vi "DistToObstNearwAng.vi"(1 "Boat Point":T1 {"North" format="%#_10f"; "East" format="%#_8f"}, 2 "Segment Point 2":T1 {"North" format="%#_10f"; "East" format="%#_8f"}, 3 "Segment Point 1":T1 {"North" format="%#_10f"; "East" format="%#_8f"}) -> (0 "Distance between boat and segment":dbl)   [LabVIEW 2012]
doc: "Takes in a segment, and a boat point, and returns the distance between the segment and the boat. For obstacle avoidance. To be added: absolute trig angle to segment."
uses:
  Data/TypeDefs/UTM Location.ctl
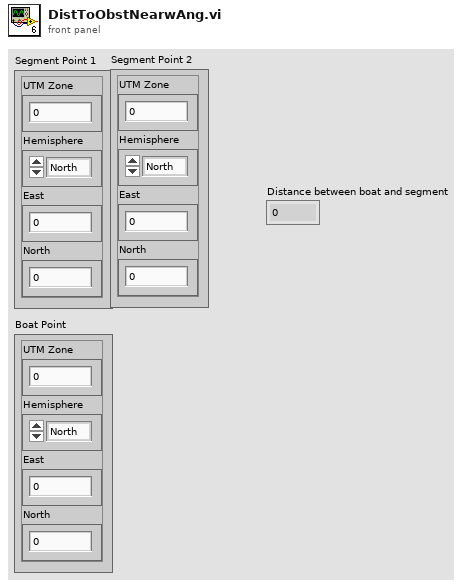
[diagram p1: front panel]
types:
  T1 = typedef "UTM Location.ctl" = cluster{"UTM Zone":dbl, "Hemisphere":enum16{"North", "South"}, "East":dbl, "North":dbl}
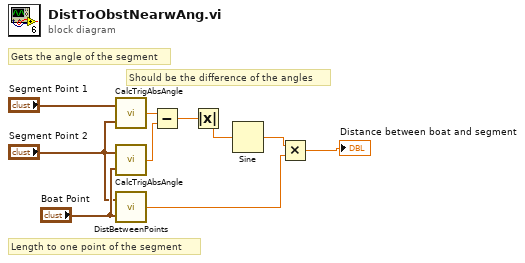
[diagram p0: block diagram]
diagram:
  # "Should be the difference of the angles"
  # "Gets the angle of the segment"
  # "Length to one point of the segment"
  n1 = call "CalcTrigAbsAngle.vi"("Point 1"="Segment Point 2", "Point 2"="Segment Point 1") -> ("Angle between points"=w7:dbl)
  n2 = call "CalcTrigAbsAngle.vi"("Point 1"="Boat Point", "Point 2"="Segment Point 2") -> ("Angle between points"=w6:dbl)
  n3 = call "DistBetweenPoints.vi"("UTM Location 2"="Boat Point", "UTM Location"="Segment Point 2") -> ("Numeric"=w4:dbl)
  n4 = Subtract(x=w7, y=w6) -> (x-y=w5:dbl)
  n5 = Absolute Value(x=w5) -> (abs(x)=w2:dbl)
  n6 = Sine(x=w2) -> (sin(x)=w1:dbl)
  n7 = Multiply(x=w1, y=w4) -> (x*y=→"Distance between boat and segment":dbl)
